vi "SVFA FFT Spectrum (Complex) (N Ch).vi"(0 "scaled signals [EU]":waveform(dbl)[](array[waveform]), 2 "window":T1=8 items=["None"=0, "Hanning"=1, "Hamming"=2, "Blackman-Harris"=3, "Exact Blackman"=4, "Blackman"=5, "Flat Top"=6, "4 Term B-Harris "=7, "7 Term B-Harris"=8, "Low Sidelobe"=9, "Force"=64, "Exponential"=65, "Blackman Nuttall"=11, "Triangle"=30, "Bartlett-Hanning"=31, "Bohman"=32, "Parzen"=33, "Welch"=34, "Kaiser"=60, "Dolph-Chebyshev"=61, "Gaussian"=62], 5 "error in (no error)":errorcluster, 7 "averaging parameters":T2={"averaging mode"=enum."No averaging", "weighting mode"=enum."Exponential", "number of averages"=10, "linear mode"=enum."One shot"} {"number of averages" min=1 step=1}, 9 "restart averaging (F)":bool) -> (11 "averaging done":bool, 13 "averages completed":dbl, 14 "complex spectra":T9(array[cluster]) {"spectrum info"."x-axis units" items=["Time (s)"=0, "Frequency-CB (Hz)"=1, "Frequency-CPB (Hz)"=1248, "Frequency-Arbitrary (Hz)"=2357, "Quefrency (s)"=2, "Revolutions (rev)"=3, "Order"=4, "Speed (RPM)"=11, "Speed (rad/s)"=21, "Index"=65535]; "spectrum info"."weighting filter" items=["Linear", "A-weighting", "B-weighting", "C-weighting", "ITU-R 468-4", "Dolby", "CCITT", "C-message", "Wb", "Wc", "Wd", "We", "Wf", "Wh", "Wj", "Wk", "Wm", "AES17 20 kHz lowpass", "AES17 40 kHz lowpass", "AES17 20 kHz highpass", "AES17 40 kHz highpass"]; "spectrum info"."dB reference [EU]" format="%.2f"; "spectrum info"."engineering units" items=["custom..."=0, "V"=1, "A"=21, "C"=30, "pC"=31, "s"=32, "-"=29, "Pa"=2, "N"=20, "g"=3, "m/s^2"=4, "m/s"=5, "m"=6, "mm/s"=12, "mm"=13, "micron/s"=14, "micron"=15, "in/s^2"=7, "in/s"=8, "in"=9, "mil/s"=10, "mil"=11, "rad/s^2"=16, "rad/s"=17, "rad"=18, "deg/s^2"=26, "deg/s"=27, "deg"=28, "RPM"=22, "cycle/s^2"=23, "Hz"=24, "cycle"=25, "strain"=19]; "spectrum info"."spectral info"."window" items=["None "=0, "Hanning"=1, "Hamming"=2, "Blackman-Harris"=3, "Exact Blackman"=4, "Blackman"=5, "Flat Top"=6, "4 Term B-Harris "=7, "7 Term B-Harris"=8, "Low Sidelobe"=9, "Force - Exponential"=10, "Gaussian"=62]; "complex spectrum response"."complex spectrum" format="%.2f"; "complex spectrum response"."df" format="%.2f"; "complex spectrum response"."f0" format="%.2f"}, 19 "error out":errorcluster)   [LabVIEW 2017]
doc: "Computes the Fast Fourier Transform (FFT) spectrum of <B>scaled signal [EU]</B>. This VI returns FFT results as the complex form of the FFT spectrum. Wire data to the <B>scaled signal [EU]</B> input to determine the polymorphic instance to use or manually select the instance."
uses:
  <vilib>/addons/_NISVFA/_Shared subVIs/Controls/svc_Spectrum Info.ctl
  <vilib>/addons/_NISVFA/_Shared subVIs/Controls/svc_X-Axis Units.ctl
  <vilib>/addons/_NISVFA/_Shared subVIs/Controls/svc_Spectrum Type.ctl
  <vilib>/addons/_NISVFA/_Shared subVIs/Controls/svc_Engineering Units Text Ring.ctl
  <vilib>/addons/_NISVFA/_Shared subVIs/Controls/svc_Weighting Filter Text Ring.ctl
  <vilib>/addons/_NISVFA/_Shared subVIs/Controls/svc_Complimentary Spectrum Units.ctl
  <vilib>/addons/_NISVFA/_Shared subVIs/Controls/svc_Window.ctl
  <vilib>/Analysis/2dsp.llb/Real FFT.vi
  <vilib>/Analysis/2dsp.llb/Power Spectrum (DBL).vi
  <vilib>/addons/_NISVFA/_Shared subVIs/Spectrum Averaging/svfa_No Average Array (complex).vi
  <vilib>/addons/_NISVFA/_Shared subVIs/Spectrum Averaging/svfa_Average Array (complex).vi
  <vilib>/addons/_NISVFA/_Shared subVIs/Common/sv_Get NI Property Name String.vi
  <vilib>/addons/_NISVFA/_Shared subVIs/Spectrum Averaging/svfa_No Average Array (real).vi
  <vilib>/addons/_NISVFA/_Shared subVIs/Spectrum Averaging/svfa_Average Array (real).vi
  <vilib>/addons/_NISVFA/_Shared subVIs/Spectrum Averaging/svfa_Peak Hold Array.vi
  <vilib>/addons/_NISVFA/_Shared subVIs/Windowing/svfa_Scaled Time Domain Window (1 Ch).vi
  <vilib>/addons/_NISVFA/_Shared subVIs/Spectrum Info/svfa_Build Spectrum Info.vi
  <vilib>/addons/_NISVFA/_Shared subVIs/Windowing/svfa_Scaled Time Domain Window (Array).vi
  <vilib>/addons/_NISVFA/_Shared subVIs/Common/svc_Get SV Channel Info.vi
  <vilib>/addons/_NISVFA/_Shared subVIs/Common/svc_Spectrum Units.vi
  <vilib>/Analysis/4window.llb/Force Window.vi
  <vilib>/Analysis/4window.llb/Force Window (DBL).vi
  <vilib>/Analysis/4window.llb/Exponential Window.vi
  <vilib>/Analysis/4window.llb/Exponential Window (DBL).vi
  <vilib>/addons/_NISVFA/_Shared subVIs/Spectrum Info/sfva_Set SV Info in Spectrum Info Description.vi
  <vilib>/addons/_NISVFA/_Shared subVIs/Spectrum Info/sfva_Get SV Info from Spectrum Info Description.vi
  <vilib>/addons/_NISVFA/_Shared subVIs/Common/svc_Get Weighting Enum and Labels.vi
  <vilib>/addons/_NISVFA/_Shared subVIs/Common/svc_Unit Label Lexical Class.vi
  <vilib>/addons/_NISVFA/_Shared subVIs/Common/svc_Engineering Units to Unit Label.vi
  <vilib>/addons/_NISVFA/_Shared subVIs/Common/svc_Format Value (DBL).vi
  <vilib>/addons/_NISVFA/_Shared subVIs/Common/svc_Channel Info to Spectrum Info.vi
  <vilib>/addons/_NISVFA/_Shared subVIs/Common/svc_Unit Label to Engineering Units.vi
  <vilib>/Utility/error.llb/Error Cluster From Error Code.vi
  <vilib>/Analysis/0measdsp.llb/Scaled Time Domain Window.vi
  <vilib>/Analysis/0measdsp.llb/Scaled Time Domain Window (DBL).vi
  <vilib>/addons/_NISVFA/_Spectrum Processing/subVIs/svfa_Spectrum Info Window to windowTd Type Def.vi
  <vilib>/addons/_NISVFA/_Shared subVIs/Common/svc_Window Parameters.vi
  <vilib>/addons/_NISVFA/_Shared subVIs/Common/svc_Get Window Info.vi
  <vilib>/Analysis/NI_AALPro.lvlib
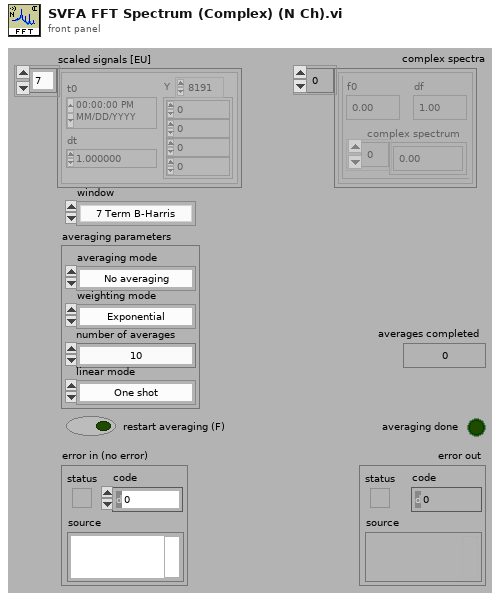
[diagram p1: front panel]
types:
  T1 = typedef "svc_Window.ctl" = u32
  T2 = cluster{"averaging mode":enum16{"No averaging", "Vector averaging", "RMS averaging", "Peak hold"}, "weighting mode":enum16{"Linear", "Exponential"}, "number of averages":u32, "linear mode":enum16{"One shot", "Auto restart"}}
  T3 = typedef "svc_Spectrum Info.ctl" = cluster{"channel name":string, "description":string, "x-axis units":T4, "spectral info":cluster{"spectrum type":T5, "linear/dB":enum16{"linear", "dB"}, "window":u16, "window size":i32, "FFT size":i32}, "engineering units":T6, "custom label":string, "dB reference [EU]":dbl, "peak units":enum16{"rms", "peak", "peak-peak"}, "weighting filter":T7, "spectral density?":bool, "unit label":string, "spectrum skewed?":bool, "complimentary spectrum units":T8}
  T4 = typedef "svc_X-Axis Units.ctl" = u16
  T5 = typedef "svc_Spectrum Type.ctl" = enum16{"FFT Spectrum [complex]", "Amplitude [Magnitude]", "Power [Magnitude^2]", "Cross Spectrum [complex]", "Frequency Response [Complex]"}
  T6 = typedef "svc_Engineering Units Text Ring.ctl" = u16
  T7 = typedef "svc_Weighting Filter Text Ring.ctl" = u16
  T8 = typedef "svc_Complimentary Spectrum Units.ctl" = enum16{"none", "radians", "degrees", "cycles", "imaginary"}
  T9 = cluster{"complex spectrum response":cluster{"f0":dbl, "df":dbl, "complex spectrum":cdb[]}, "spectrum info":T3}[]
  T10 = enum16{"Restart processing", "Continue processing", "Skip processing"}
  T11 = cluster{"complex FFT":cdb[], "real FFT":dbl[], "f0":dbl, "df":dbl, "averages completed":dbl, "averaging parameters":cluster{"averaging mode":enum16{"No averaging", "Vector averaging", "RMS averaging", "Peak hold"}, "weighting mode":enum16{"Linear", "Exponential"}, "number of averages":u32, "linear mode":enum16{"One shot", "Auto restart"}}}[]
  T12 = cluster{"complex spectrum response":cluster{"f0":dbl, "df":dbl, "complex spectrum":cdb[]}, "spectrum info":T3}
  T13 = enum16{"No averaging", "Vector averaging", "RMS averaging", "Peak hold"}
  T14 = cluster{"complex FFT":cdb[], "real FFT":dbl[], "f0":dbl, "df":dbl, "averages completed":dbl, "averaging parameters":cluster{"averaging mode":enum16{"No averaging", "Vector averaging", "RMS averaging", "Peak hold"}, "weighting mode":enum16{"Linear", "Exponential"}, "number of averages":u32, "linear mode":enum16{"One shot", "Auto restart"}}}
  T15 = cluster{"complex FFT":cdb[], "Mag/Real FFT":dbl[], "f0":dbl, "df":dbl, "averages completed":dbl, "averaging parameters":cluster{"averaging mode":enum16{"No averaging", "Vector averaging", "RMS averaging", "Peak hold"}, "weighting mode":enum16{"Linear", "Exponential"}, "number of averages":u32, "linear mode":enum16{"One shot", "Auto restart"}}}
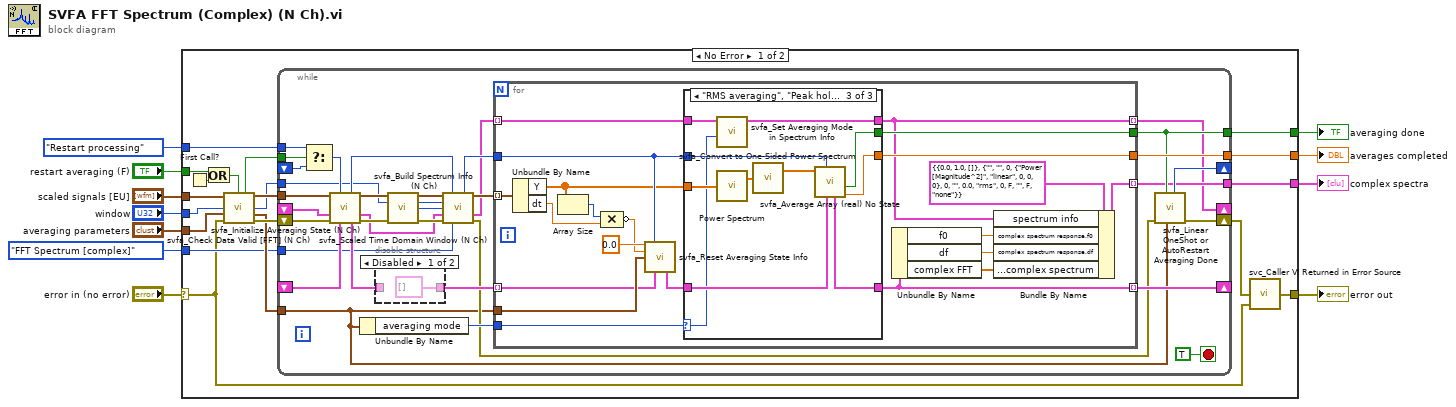
[diagram p0: block diagram]
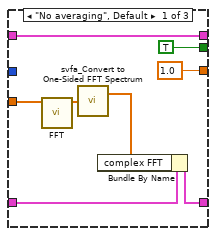
[diagram p3: hidden frame]
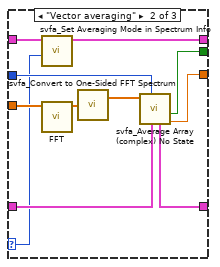
[diagram p4: hidden frame]
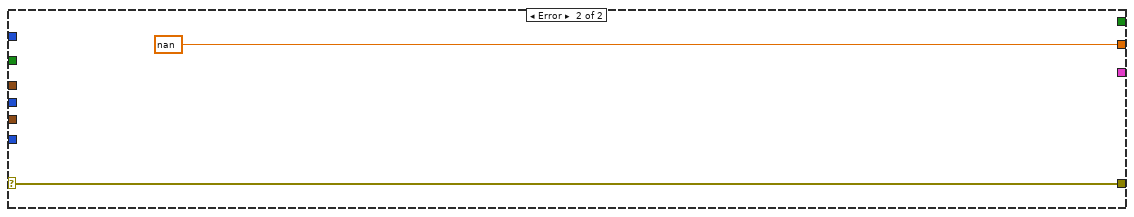
[diagram p5: hidden frame]
diagram:
  n1 = case shown="No Error" "error in (no error)" {
    selector: "error in (no error)" -> [w13 w118]
    tunnel: "scaled signals [EU]" -> [w30 _]
    tunnel: "averaging parameters" -> [w29 _]
    tunnel: [w27 w118] -> w8
    tunnel: [w24 _] -> w7
    tunnel: [w23 nan ("averages completed")] -> w6
    tunnel: "window" -> [w28 _]
    tunnel: [w12 _] -> w4
    tunnel: T10."Restart processing" ("t") -> [w18 _]
    tunnel: svc_Spectrum_Type."FFT Spectrum [complex]" ("spectrum type") -> [w17 _]
    tunnel: "restart averaging (F)" -> [w15 _]
    frame No Error {
      n2 = First Call?() -> (First Call?: T/F=w16:bool)
      n3 = Or(x=w15, y=w16) -> (x .or. y?=w14:bool)
      n4 = call <vilib>:"svfa_Check Data Valid [FFT] (N Ch).vi"("scaled signals"=w30, "restart averaging (F)"=w14, "window"=w28, "averaging parameters"=w29, "error in (no error)"=w13) -> ("restart averaging"=w19:bool, "dup scaled signals"=w26:waveform(dbl)[], "dup window"=w21:T1, "dup averaging parameters"=w20:T2, "error out"=w25:errorcluster)  [unwired: 6 in]
      n5 = while {
        tunnel: [w62] -> w23
        tunnel: [w58] -> w24
        shift-left: _ -> [w59]
        shift-right: [w60] -> _
        shift-right: [w32] -> _
        shift-left: _ -> [w55]
        tunnel: w21 -> [w35]
        tunnel: w20 -> [w31]
        tunnel: w18 -> [w54]
        tunnel: w19 -> [w53]
        shift-right: [w57] -> _
        shift-left: _ -> [w52]
        tunnel: w17 -> [w37]
        shift-right: [w56] -> w22
        shift-left: w25 -> [w61]
        tunnel: w26 -> [w63]
        tunnel: [w34] -> w12
        stop <- TRUE stop-if-true
        n6 = Select(t=w54, s=w53, f=w52) -> (s? t:f=w51:T10)
        n7 = call <vilib>:"svfa_Initialize Averaging State (N Ch).vi"("Windowed Waveform(s)"=w63, "processing control in"=w51, "spectra info in"=w55, "error in (no error)"=w61, "state info"=w59) -> ("processing control out"=w42:T10, "Windowed Waveform(s)"=w50:waveform(dbl)[], "spectra info out"=w43:T3[], "state info"=w39:T11, "error out"=w49:errorcluster)  [unwired: 6 in]
        n8 = Unbundle By Name(w31) -> ("averaging mode"=w44:T13)
        n9 = disable-structure shown="Disabled" {
          disable-tunnel: [T11 [] ("state info") w66] -> w38
          disable-tunnel: w39 -> [_ w66]
          frame Disabled {
          }
          frame Enabled {
          }
        }
        n10 = call <vilib>:"svfa_Scaled Time Domain Window (N Ch).vi"("Scaled signal(s)"=w50, "window"=w35, "error in (no error)"=w49) -> ("Windowed Waveform(s)"=w48:waveform(dbl)[], "window"=w47:T1, "window length"=w41:i32, "error out"=w46:errorcluster)  [unwired: 8 in, 1 out]
        n11 = call <vilib>:"svfa_Build Spectrum Info (N Ch).vi"("scaled signal(s)"=w48, "processing control in"=w42, "window"=w47, "window size"=w41, "spectra info in"=w43, "error in (no error)"=w46, "spectrum type"=w37) -> ("dup processing control"=w45:T10, "dup scaled signals"=w40:waveform(dbl)[], "spectra info out"=w33:T3[], "error out"=w36:errorcluster)  [unwired: 5 in]
        n12 = for {
          tunnel: w45 -> [w83]
          tunnel: w38 -> [w79] mode=indexing
          tunnel: [w86] -> w58
          tunnel: [w87] -> w62
          tunnel: w40 -> [w84] mode=indexing
          tunnel: w31 -> [w81]
          tunnel: [w69] -> w60 mode=indexing
          tunnel: w44 -> [w85]
          tunnel: [w70] -> w34 mode=indexing
          tunnel: w33 -> [w68] mode=indexing
          tunnel: [w67] -> w32 mode=indexing
          n13 = Unbundle By Name ("Get Waveform Components")(w84) -> ("Y"=w77:dbl[], "dt"=w80:dbl)
          n14 = Array Size(array=w77) -> (size(s)=w75:i32)
          n15 = Compound Arithmetic op=MULTIPLY(w75, w80) -> (invert w76:dbl)
          n16 = call <vilib>:"svfa_Reset Averaging State Info.vi"("f0"=0.0, "processing control"=w83, "df"=w76, "averaging parameters"=w81, "averaging state info in"=w79) -> ("averaging state info out"=w78:T14)  [unwired: 9 in, 1 out]
          n17 = case shown="\"RMS averaging\", \"Peak hold\"" w85 {
            selector: w85 -> [_ w96 w107]
            tunnel: w83 -> [_ w106 w114]
            tunnel: w78 -> [w93 w105 w117]
            tunnel: w77 -> [w90 w101 w112]
            tunnel: [TRUE ("averaging done") w104 w115] -> w86
            tunnel: [1.0 ("averages completed") w103 w116] -> w87
            tunnel: [w92 w99 w110] -> w69
            tunnel: w68 -> [w88 w98 w109]
            tunnel: [w88 w97 w108] -> w67
            frame "No averaging", Default {
              n18 = call-poly <vilib>:"FFT.vi"("X"=w90) -> ("FFT {X}"=w91:cdb[])  [unwired: 9 in, 1 out]
              n19 = call <vilib>:"svfa_Convert to One-Sided FFT Spectrum.vi"("two-sided FFT spectrum"=w91) -> ("one-sided FFT spectrum"=w89:cdb[])  [unwired: 1 out]
              n20 = Bundle By Name(cluster=w93, "complex FFT"=w89) -> (w92:T14)
            }
            frame "Vector averaging" {
              n21 = call <vilib>:"svfa_Set Averaging Mode in Spectrum Info.vi"("averaging mode"=w96, "spectrum info in"=w98) -> ("spectrum info out"=w97:T3)  [unwired: 8 in, 1 out]
              n22 = call-poly <vilib>:"FFT.vi"("X"=w101) -> ("FFT {X}"=w102:cdb[])  [unwired: 9 in, 1 out]
              n23 = call <vilib>:"svfa_Convert to One-Sided FFT Spectrum.vi"("two-sided FFT spectrum"=w102) -> ("one-sided FFT spectrum"=w100:cdb[])  [unwired: 1 out]
              n24 = call <vilib>:"svfa_Average Array (complex) No State.vi"("averaging state info in"=w105, "processing control"=w106, "array"=w100) -> ("averages completed"=w103:dbl, "averaging done"=w104:bool, "averaging state info out"=w99:T15)  [unwired: 5 in, 1 out]
            }
            frame "RMS averaging", "Peak hold" {
              n25 = call <vilib>:"svfa_Set Averaging Mode in Spectrum Info.vi"("averaging mode"=w107, "spectrum info in"=w109) -> ("spectrum info out"=w108:T3)  [unwired: 8 in, 1 out]
              n26 = call-poly <vilib>:"Power Spectrum.vi"("X"=w112) -> ("Power Spectrum"=w113:dbl[])  [unwired: 1 out]
              n27 = call <vilib>:"svfa_Convert to One-Sided Power Spectrum.vi"("two-sided power spectrum"=w113) -> ("one-sided power spectrum"=w111:dbl[])  [unwired: 1 out]
              n28 = call <vilib>:"svfa_Average Array (real) No State.vi"("averaging state info in"=w117, "processing control"=w114, "array"=w111) -> ("averages completed"=w116:dbl, "averaging done"=w115:bool, "averaging state info out"=w110:T15)  [unwired: 5 in, 1 out]
            }
          }
          n29 = Unbundle By Name(w69) -> ("f0"=w72:dbl, "df"=w73:dbl, "complex FFT"=w74:cdb[])
          n30 = Bundle By Name(cluster=T12 {"complex spectrum response"={"f0"=0.0, "df"=1.0, "complex spectrum"=[]}, "spectrum info"={"channel name"="", "description"="", "x-axis units"=0, "spectral info"={"spectrum type"=enum."Power [Magnitude^2]", "linear/dB"=enum."linear", "window"=0, "window size"=0, "FFT size"=0}, "engineering units"=0, "custom label"="", "dB reference [EU]"=0.0, "peak units"=enum."rms", "weighting filter"=0, "spectral density?"=FALSE, "unit label"="", "spectrum skewed?"=FALSE, "complimentary spectrum units"=enum."none"}} ("complex spectrum"), "spectrum info"=w67, "complex spectrum response.f0"=w72, "complex spectrum response.df"=w73, "complex spectrum response.complex spectrum"=w74) -> (w70:T12)
        }
        n31 = call <vilib>:"svfa_Linear OneShot or AutoRestart Averaging Done.vi"("averaging parameters"=w31, "averaging done"=w58, "error in (no error)"=w36) -> ("error out"=w56:errorcluster, "processing control"=w57:T10)  [unwired: 7 in]
      }
      n32 = call <vilib>:"svc_Caller VI Returned in Error Source.vi"("warning input to caller"=w13, "error in (no error)"=w22) -> ("error out"=w27:errorcluster)  [unwired: 3 in]
    }
    frame Error {
    }
  }
  "error out" <- w8
  "averaging done" <- w7
  "averages completed" <- w6
  "complex spectra" <- w4
